vi "Reinitial Parameter After Test.vi"(8 "error in (no error)":errorcluster, 11 "main ref":T1) -> (0 "error out":errorcluster)   [LabVIEW 2025]
uses:
  controls/LAB-IQ UI Data.ctl
  Traction Loop/Traction Receipe Enum.ctl
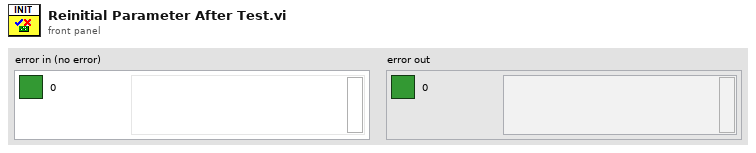
[diagram p1: front panel]
types:
  T1 = typedef "LAB-IQ UI Data.ctl" = cluster{"Main Home Screen":cluster{"GUI":refnum<vi>, "Platform Settings":refnum<vi>, "Configure":refnum<vi>, "Home":refnum<vi>, "EXIT":refnum<vi>, "service 2":refnum<vi>, "MainPage":refnum<vi>, "Analysis":refnum<vi>}, "Platform Settings":cluster{"mm/s  Surge":refnum<vi>, "Drive Error":refnum<vi>, "Disable Axis Jog Soft Limits":refnum<vi>, "mm/s  Sway":refnum<vi>, "Sway and Surge COM Status":refnum<vi>, "Heave COM Status":refnum<vi>, "Enable Platform":refnum<vi>, "Surge Forward Main":refnum<vi>, "Sway Right Main":refnum<vi>, "Sway Left Main":refnum<vi>, "Heave Down Main":refnum<vi>, "Heave Up main":refnum<vi>, "mm/s Heave":refnum<vi>, "mm/sec":refnum<vi>, "mm":refnum<vi>, "Surge Backward Main":refnum<vi>}, "Analysis Screen":cluster{"Analysis Home":refnum<vi>, "Surface Analysis":refnum<vi>, "Imaging":refnum<vi>, "Image Analysis":refnum<vi>, "Post Analysis":refnum<vi>}, "Config Screen":cluster{"Select Load Head":refnum<vi>, "Notes :":refnum<vi>, "FILE":refnum<vi>, "Sample ID :":refnum<vi>, "Operator ID :":refnum<vi>, "Operator Name :":refnum<vi>, "Auto":refnum<vi>}, "Motion Module":cluster{"zNL":refnum<vi>, "NL disp":refnum<vi>, "Rotary Tab":refnum<vi>, "Motion Direction:  3":refnum<vi>, "E.Velocity 2":refnum<vi>, "e.v/ssr 2":refnum<vi>, "Enter Fixed E.Velocity 2":refnum<vi>, "Enter Final SRR 2":refnum<vi>, "Enter initial SRR 2":refnum<vi>, "Enter Fixed SRR 2":refnum<vi>, "Enter the Final E.Velocity (m/s) 2":refnum<vi>, "Enter initial E.Velocity (m/s) 2":refnum<vi>, "Final Speed (RPM) 3":refnum<vi>, "Initial Speed (RPM) 2":refnum<vi>, "Enter the Final Velocity (m/s) 3":refnum<vi>, "Enter initial Velocity (m/s)  3":refnum<vi>, "Ramp Up 2":refnum<vi>, "TEST SELECTION":refnum<vi>, "SPEED SELECTION : ":refnum<vi>, "Angular Oscillation Set":refnum<vi>, "Traction":refnum<vi>, "Step Speed":refnum<vi>, "StepTable For Load-Speed":refnum<vi>, "StepTable For Speed":refnum<vi>, "Surge Forward MM":refnum<vi>, "Surge Backward MM":refnum<vi>, "M3 Image":refnum<vi>, "String 39":refnum<vi>, "Sway Left MM":refnum<vi>, "Sway Right MM":refnum<vi>, "Disable Axis Jog Soft Limits":refnum<vi>, "mm":refnum<vi>, "Heave Down MM":refnum<vi>, "Heave Up MM":refnum<vi>, "Wear Track Diameter (mm)":refnum<vi>, "Set WTD":refnum<vi>, "HomeScratch":refnum<vi>, "HomeRot":refnum<vi>, "PlaceModule":refnum<vi>, "Enter the Angle (Deg)":refnum<vi>, "Enter the Frequency (Hz)":refnum<vi>, "Motion Mode:":refnum<vi>, "LR Sway":refnum<vi>, "Rot Hor":refnum<vi>, "Scratch":refnum<vi>, "LR Cam":refnum<vi>, "MMBack":refnum<vi>, "MMNext":refnum<vi>, "Rot Ver":refnum<vi>, "Rotary Module Selection":refnum<vi>, "calculate rotary":refnum<vi>, "SPEED SELECTION : rotary":refnum<vi>, "Import 2":refnum<vi>, "Save 2":refnum<vi>, "File Path :  2":refnum<vi>, "String 45":refnum<vi>, "StepTable For Speed 3":refnum<vi>, "Enter the Speed(mm/sec)":refnum<vi>, "Enter the Speed(RPM)":refnum<vi>, "Enter Scratch Speed (mm/s):":refnum<vi>, "SwaySpeed Set":refnum<vi>, "Scartch Offset":refnum<vi>, "Motion type:":refnum<vi>, "HomeScratch 2":refnum<vi>, "Enter Scratch length (mm):":refnum<vi>, "Wear Track Diameter":refnum<vi>, "Rotary Speed Exced":refnum<vi>, "Scratch Mode":refnum<vi>, "No of Scratch":refnum<vi>}, "Environmental control":cluster{"Humidity  Status  3":refnum<vi>, "Low Temp  Status  2":refnum<vi>, "TK4 status 2":refnum<vi>, "Stage Temperature":refnum<vi>, "Sample Temperature":refnum<vi>, "Humidity (Amb)":refnum<vi>, "Clear List":refnum<vi>, "Add to list":refnum<vi>, "Wear":refnum<vi>, "Vibration":refnum<vi>, "Humidity (Chamber)":refnum<vi>, "Temperature (Chamber)":refnum<vi>, "ECR ":refnum<vi>, "Temperature (Amb)":refnum<vi>, "Microphone":refnum<vi>, "Acoustic Emission 3":refnum<vi>, "SNext":refnum<vi>, "APBack":refnum<vi>, "Enter the Temperature (°C):":refnum<vi>, "Enter the Stage \nTemperature (°C):":refnum<vi>, "Enter the Humidity (%Rh):":refnum<vi>, "Low Temp":refnum<vi>, "High Temp":refnum<vi>, "Humidity":refnum<vi>, "Sensors Picked":refnum<vi>}, "About Screen":cluster{"Password":refnum<vi>, "Home Service":refnum<vi>, "Advanced Setting":refnum<vi>, "About Tab":refnum<vi>, "ECR Port:":refnum<vi>, "Ramp Port:":refnum<vi>, "Installation/Replacement completed":refnum<vi>, "Loahead":refnum<vi>, "Heave and Surge COM Port:":refnum<vi>, "Sway COM Port:":refnum<vi>, "Temp Modbus:":refnum<vi>, "Humidity Port:":refnum<vi>, "Edit Gain Constants":refnum<vi>, "Save Gain Constants":refnum<vi>}, "Main Screen":cluster{"Main Screen Tab":refnum<vi>, "Angle and Frequency":refnum<vi>, "Stroke (mm)":refnum<vi>, "Angle (Deg)":refnum<vi>, "Main Speed Tab":refnum<vi>, "MTM MOTOR DISPLAY":refnum<vi>, "Disc Speed (m/sec)":refnum<vi>, "Ball Speed (m/sec)":refnum<vi>, "Disc Speed (RPM)":refnum<vi>, "Ball Speed (RPM)":refnum<vi>, "SPEED TAB":refnum<vi>, "Speed (m/sec)":refnum<vi>, "Set Speed (m/sec)":refnum<vi>, "Speed (RPM)":refnum<vi>, "Set Speed":refnum<vi>, "Time Tab":refnum<vi>, "Time ( HH:MM:SS ) 2":refnum<vi>, "Test Duration":refnum<vi>, "Test Duration 4":refnum<vi>, "TEST CYCLE":refnum<vi>, "TOTAL CYCLES":refnum<vi>, "Set Load (N)":refnum<vi>, "Temp Tabs":refnum<vi>, "Heater":refnum<vi>, "TK4 status":refnum<vi>, "ChamberTemp":refnum<vi>, "SetTmp":refnum<vi>, "Controller  Status":refnum<vi>, "ChamberTemp 2":refnum<vi>, "SetTmp 2":refnum<vi>, "Controller  Status 2":refnum<vi>, "ChamberTemp 3":refnum<vi>, "SetTmp 3":refnum<vi>, "Cooling":refnum<vi>, "Load Communication":refnum<vi>, "Ambient \nTemperature":refnum<vi>, "HumCOMStatus":refnum<vi>, "Ambient\n Humidity":refnum<vi>, "Freq (Hz)":refnum<vi>, "Load En":refnum<vi>, "NLt":refnum<vi>, "zNL 2":refnum<vi>, "Humidity On":refnum<vi>, "humidity disp":refnum<vi>, "Set Humidity":refnum<vi>, "NL disp 2":refnum<vi>, "Humidity On 2":refnum<vi>, "humidity disp 2":refnum<vi>, "Set Humidity 2":refnum<vi>, "NL disp 3":refnum<vi>, "AppLoadSeq scratch":refnum<vi>, "Stop Scratch":refnum<vi>, "ClrLog":refnum<vi>, "Trip Log":refnum<vi>, "STOP":refnum<vi>, "Start Test":refnum<vi>, "Test status":refnum<vi>, "AR Led":refnum<vi>, "Data":refnum<vi>, "Health":refnum<vi>, "Sway COM Status":refnum<vi>, "Heave COM Status":refnum<vi>, "Grp Tab":refnum<vi>, "Sub Graph":refnum<vi>, "SD (mm)":refnum<vi>, "Siliding distance Reset Graph":refnum<vi>, "SDGp":refnum<vi>, "Humidity Reset Graph":refnum<vi>, "HumrGp":refnum<vi>, "Acoustic Emission (mV)":refnum<vi>, "Aqucostic Reset Graph":refnum<vi>, "gACQUOS":refnum<vi>, "ECR RESET":refnum<vi>, "ECR":refnum<vi>, "Temperature Reset":refnum<vi>, "Acoustic Emission (mV) 2":refnum<vi>, "Aqucostic Reset Graph 2":refnum<vi>, "gACQUOS 2":refnum<vi>, "ECR RESET 2":refnum<vi>, "ECR 2":refnum<vi>, "Temperature Reset 2":refnum<vi>, "Temperature (deg c)":refnum<vi>, "Speed Reset Graph":refnum<vi>, "Speed Tab":refnum<vi>, "MTM DISC  SPEED":refnum<vi>, "MTM BALL SPEED":refnum<vi>, "speed mm/sec":refnum<vi>, "Hymidity":refnum<vi>, "Humidity Disable trip":refnum<vi>, "CoF Trip  2":refnum<vi>, "Depth Trip":refnum<vi>, "Weart Deapth":refnum<vi>, "Depth Reset Graph":refnum<vi>, "Weart":refnum<vi>, "Depthz":refnum<vi>, "Depth (µm)":refnum<vi>, "WearGp":refnum<vi>, "NL Trip 2":refnum<vi>, "Load pid":refnum<vi>, "Load Disable Trip":refnum<vi>, "Load Reset Graph":refnum<vi>, "NL Display 4":refnum<vi>, "Main Chart 3":refnum<vi>, "BACK":refnum<vi>, "Depth Trip 2":refnum<vi>, "COF TRIP ":refnum<vi>, "Friction Force (N)":refnum<vi>, "FF Reset Graph":refnum<vi>, "FF Disable Trip":refnum<vi>, "FF TRIP":refnum<vi>, "COF Disable Trip":refnum<vi>, "COF Reset Graph":refnum<vi>, "Start Test Temp":refnum<vi>, "zFF":refnum<vi>, "Friction Force (N) Graph":refnum<vi>, "Coefficient of Friction":refnum<vi>, "Scratch Start Test":refnum<vi>, "FF Tab":refnum<vi>, "Cyclic Friction Force (N)":refnum<vi>, "CZ FF":refnum<vi>, "Cyclic Friction Force (N) Graph":refnum<vi>, "Cyclic Coefficient of Friction":refnum<vi>, "Cyclic FF TRIP":refnum<vi>, "Cyclic FF Disable Trip":refnum<vi>, "cyclic COF Disable Trip":refnum<vi>, "cyclic COF TRIP":refnum<vi>, "cyclic COF Reset Graph":refnum<vi>, "Cyclic FF Reset Graph":refnum<vi>, "Test Trip":refnum<vi>, "Multi Scratch Pass":refnum<vi>, "Scratch Start Recording":refnum<vi>}, "Loading":cluster{"Indentation":refnum<vi>, "Reference Sample":refnum<vi>, "Load Cell Communication Slide":refnum<vi>, "com 3":refnum<vi>, "com":refnum<vi>, "DecaForce COM Status":refnum<vi>, "Update":refnum<vi>, "Clear 3":refnum<vi>, "seq":refnum<vi>, "Stribeck table":refnum<vi>, "Stribeck Table  For loading":refnum<vi>, "Loading Mode":refnum<vi>, "Enter the Final Load (N)":refnum<vi>, "Enter the CoF Trip":refnum<vi>, "Enter the Friction Force Trip":refnum<vi>, "Enter the Normal load Trip":refnum<vi>, "Enter the Load  (N)":refnum<vi>, "KiloForce":refnum<vi>, "DecaForce ":refnum<vi>, "MicroForce":refnum<vi>, "LHBack":refnum<vi>, "LHNext":refnum<vi>, "Enter the Loading Rate (N/min)":refnum<vi>, "Message":refnum<vi>, "Warning 2":refnum<vi>, "SSP 0.75":refnum<vi>, "SSP 0.5":refnum<vi>, "SSP 0.3":refnum<vi>, "Warning":refnum<vi>, "gui GIF":refnum<vi>, "Communication is established":refnum<vi>, "AppLoad 4":refnum<vi>, "Multipoint":refnum<vi>, "Load Selection":refnum<vi>}, "PID":cluster{"Ramp":refnum<vi>, "Vertical load (N)":refnum<vi>, "apply load":refnum<vi>, "apply load 2":refnum<vi>, "Enter ByPass Load":refnum<vi>, "Bypass Load":refnum<vi>, "gFF Rot":refnum<vi>}, "Config Parameters":cluster{"Tab Control 3":refnum<vi>, "Tab Control 19":refnum<vi>, "SAMPLES":refnum<vi>, "Re-initilaize":refnum<vi>, "Filter ON/OFF":refnum<vi>, "TracHomeSurgeOffsetCounts 10MM":refnum<vi>, "TracHomeSwayOffsetCounts 10MM":refnum<vi>, "Acoustic Emission:":refnum<vi>, "Apply Filter (FF)":refnum<vi>, "Filter% 2":refnum<vi>, "Apply Filter (Load)":refnum<vi>, "Filter% ":refnum<vi>, "Sway distance (mm)":refnum<vi>, "Surge distance (mm)":refnum<vi>, "DataSavingLoopDelay(ms)":refnum<vi>, "SAVE 2":refnum<vi>, "Enter Distance":refnum<vi>, "Sway Counts:":refnum<vi>, "Distance (mm): 3":refnum<vi>, "Surge Counts:":refnum<vi>, "Distance (mm): 2":refnum<vi>, "Distance (mm):":refnum<vi>, "Heave Counts:":refnum<vi>, "LRMHomeSurgeOffsetCounts":refnum<vi>, "LRMHomeSwayOffsetCounts":refnum<vi>, "TracHomeSurgeOffsetCounts 20MM":refnum<vi>, "TracHomeSwayOffsetCounts 20MM":refnum<vi>, "RotHomeSwayOffsetCounts":refnum<vi>, "RotHomeSurgeOffsetCounts":refnum<vi>, "Heave distance":refnum<vi>, "Zmm":refnum<vi>, "Heave Pulses/mm":refnum<vi>, "Surge Pulses/mm":refnum<vi>, "Sway Pulses/mm":refnum<vi>, "Heave Pitch":refnum<vi>, "Surge Pitch":refnum<vi>, "Sway Pitch":refnum<vi>, "Heave PPR":refnum<vi>, "Surge PPR":refnum<vi>, "Sway PPR":refnum<vi>, "Tab Control 5":refnum<vi>, "Tab Control 14":refnum<vi>, "Tab Control 26":refnum<vi>, "AE":refnum<vi>, "Heave Loop Delay":refnum<vi>, "Heave PID Speed":refnum<vi>, "Surge Jog Speed":refnum<vi>, "Heave Jog Speed":refnum<vi>, "Sway Loop Delay":refnum<vi>, "Sway PID Speed":refnum<vi>, "Sway Jog Speed":refnum<vi>, "DEPTH TRIP VALUE":refnum<vi>, "LOAD TRIP VALUE":refnum<vi>, "DEPTH TRIP   ENABLE":refnum<vi>, "LOAD TRIP  ENABLE":refnum<vi>, "CYCLIC FF TRIP VALUE":refnum<vi>, "FF TRIP VALUE":refnum<vi>, "CYCLIC CoF TRIP VALUE":refnum<vi>, "COF TRIP VALUE":refnum<vi>, "CYCLIC COF TRIP  ENABLE":refnum<vi>, "CYCLIC FF TRIP  ENABLE":refnum<vi>, "FF TRIP  ENABLE":refnum<vi>, "COF TRIP  ENABLE":refnum<vi>, "JOG TRIP LOAD VALUE (N)":refnum<vi>, "Rotary Vertical":refnum<vi>, "Traction":refnum<vi>, "Scratch":refnum<vi>, "LRM CAM":refnum<vi>, "Sway LRM":refnum<vi>, "Rotary Horizontal":refnum<vi>}, "Loading Com Port":cluster{"ClearAll":refnum<vi>, "Mz(Nm)":refnum<vi>, "My(Nm)":refnum<vi>, "Mx(Nm)":refnum<vi>, "Save Dwell":refnum<vi>, "Acq Delay (ms)":refnum<vi>, "Burst Delay (ms)":refnum<vi>, "model":refnum<vi>, "SN":refnum<vi>, "FFx(N)":refnum<vi>, "Sensor IP":refnum<vi>, "Port":refnum<vi>, "FFy(N)":refnum<vi>, "Load(N)":refnum<vi>, "delete Handle":refnum<vi>, "Create Handle":refnum<vi>, "ft_data":refnum<vi>, "ft_range":refnum<vi>, "ft_data 2":refnum<vi>, "stop 6":refnum<vi>, "running_flag":refnum<vi>, "ft_udp_handle":refnum<vi>, "get-data-return":refnum<vi>, "get-range-return":refnum<vi>, "zero-return":refnum<vi>, "filter-return":refnum<vi>, "initial-return":refnum<vi>, "deleteHandle-result":refnum<vi>, "Load Cell Temp":refnum<vi>, "Load Cell":refnum<vi>, "ZeroAll":refnum<vi>, "FORCE (N)":refnum<vi>, "TORQUE (N-m)":refnum<vi>, "Load Cell Link":refnum<vi>}, "Heave AND Surge":cluster{"SURGE POSE":refnum<vi>, "error out Read":refnum<vi>, "HEAVE POSE":refnum<vi>, "State":refnum<vi>, "Homed":refnum<vi>, "Sequence ID":refnum<vi>, "error out Write":refnum<vi>, "faultCode":refnum<vi>, "Ack ID":refnum<vi>, "SPEED":refnum<vi>, "Distance":refnum<vi>, "Mode Command":refnum<vi>, "Heave and Surge Read":refnum<vi>, "Read Heave Temp":refnum<vi>, "Spare 15":refnum<vi>, "Spare 14":refnum<vi>, "Spare 13":refnum<vi>, "Spare 12":refnum<vi>, "Spare 11":refnum<vi>, "Spare 10":refnum<vi>, "Spare 9":refnum<vi>, "Spare 8":refnum<vi>, "Spare 7":refnum<vi>, "Spare 4":refnum<vi>, "Spare 3":refnum<vi>, "Spare 2":refnum<vi>, "Humidity":refnum<vi>, "Temp":refnum<vi>, "Node Id":refnum<vi>, "Spare 1":refnum<vi>, "SPARE 4":refnum<vi>, "SPARE 3":refnum<vi>, "SPARE 2":refnum<vi>, "SPARE 1":refnum<vi>, "fwMajor":refnum<vi>, "fwMinor":refnum<vi>, "Manual Write":refnum<vi>, "Heave and Surge Write":refnum<vi>, "SPARE 5":refnum<vi>, "Reserved ":refnum<vi>, "SPARE 8":refnum<vi>, "SPARE 6":refnum<vi>, "SPARE 7":refnum<vi>, "SPARE 17":refnum<vi>, "SPARE 16":refnum<vi>, "SPARE 15":refnum<vi>, "SPARE 14":refnum<vi>, "SPARE 13":refnum<vi>, "SPARE 12":refnum<vi>, "SPARE 11":refnum<vi>, "SPARE 10":refnum<vi>, "SPARE 9":refnum<vi>, "System UPTIME":refnum<vi>, "Missed Packets":refnum<vi>, "faultCode Surge Right":refnum<vi>, "faultCode Surge Left":refnum<vi>, "faultCode Heave":refnum<vi>, "UPLINK HEAVE":refnum<vi>, "DOWNLINK HEAVE":refnum<vi>}, "New PID LOGIC":cluster{"Fine Tune Zone":refnum<vi>, "PID SDelay":refnum<vi>, "Max_pos_limit":refnum<vi>, "Min_pos_limit":refnum<vi>, "i_limit":refnum<vi>, "pct_scale":refnum<vi>, "Deadband":refnum<vi>, "Kd":refnum<vi>, "Ki":refnum<vi>, "Kp":refnum<vi>, "Current Position":refnum<vi>, "Set Load":refnum<vi>, "Current Load":refnum<vi>, "Pulse delta":refnum<vi>, "Init Step":refnum<vi>, "Max Step Linit":refnum<vi>, "min_deadband_floor":refnum<vi>, "dynamic_spindle_noise_scalar":refnum<vi>, "min_finetune_floor":refnum<vi>, "filter_alpha":refnum<vi>, "PID":refnum<vi>}, "SWAY ":cluster{"fwMajor":refnum<vi>, "Homed":refnum<vi>, "Rotary POSE":refnum<vi>, "State":refnum<vi>, "SWAY POSE":refnum<vi>, "Ack ID":refnum<vi>, "faultCode":refnum<vi>, "Node Id":refnum<vi>, "fwMinor":refnum<vi>, "Spare 6":refnum<vi>, "Spare 5":refnum<vi>, "Spare 4":refnum<vi>, "Spare 3":refnum<vi>, "Spare 2":refnum<vi>, "Spare 1":refnum<vi>, "Spare 7":refnum<vi>, "SPARE  5":refnum<vi>, "error out Write  SWAY ":refnum<vi>, "error out Read SWAY ":refnum<vi>, "Manual Write SWAY ":refnum<vi>, "SWAY WRITE":refnum<vi>, "SPARE  4":refnum<vi>, "SPARE  3":refnum<vi>, "SPARE 2":refnum<vi>, "SPARE 1":refnum<vi>, "Spare 15":refnum<vi>, "Spare 14":refnum<vi>, "Spare 13":refnum<vi>, "Spare 12":refnum<vi>, "Spare 11":refnum<vi>, "Spare 9":refnum<vi>, "Spare 8":refnum<vi>, "SPEED":refnum<vi>, "Distance":refnum<vi>, "Mode Command":refnum<vi>, "Sequence ID":refnum<vi>, "SWAY READ":refnum<vi>, "Spare 10":refnum<vi>, "Read SWAY Temp":refnum<vi>, "faultCode Sway ":refnum<vi>, "Missed Packets":refnum<vi>, "System UPTIME sway":refnum<vi>, "SPARE 6":refnum<vi>, "SPARE 7":refnum<vi>, "SPARE 9":refnum<vi>, "SPARE 11":refnum<vi>, "SPARE 10":refnum<vi>, "SPARE 8":refnum<vi>, "SPARE 13":refnum<vi>, "SPARE 12":refnum<vi>, "SPARE 17":refnum<vi>, "SPARE 16":refnum<vi>, "SPARE 15":refnum<vi>, "SPARE 14":refnum<vi>, "Reserved":refnum<vi>, "faultCode Rotary":refnum<vi>, "UPLINK SWAY":refnum<vi>, "DOWNLINK SWAY":refnum<vi>}, "Analysis Screen":cluster{"Analysis Home":refnum<vi>, "Refresh 2":refnum<vi>, "MEAN 4":refnum<vi>, "SD 4":refnum<vi>, "VARIANCE 4":refnum<vi>, "MEAN  3":refnum<vi>, "SD  3":refnum<vi>, "VARIANCE  3":refnum<vi>, "MEAN 2":refnum<vi>, "SD  2":refnum<vi>, "VARIANCE 2":refnum<vi>, "MEAN":refnum<vi>, "SD":refnum<vi>, "VARIANCE":refnum<vi>, "File 4 Discription":refnum<vi>, "OPEN 4":refnum<vi>, "File Name 4":refnum<vi>, "OPEN 3":refnum<vi>, "File 3 Discription":refnum<vi>, "File Name 3":refnum<vi>, "Y-AXIS":refnum<vi>, "X-AXIS":refnum<vi>, "XY Graph":refnum<vi>, "File Name 2":refnum<vi>, "File Name 1":refnum<vi>, "OPEN 2":refnum<vi>, "OPEN 1":refnum<vi>, "File 1 Discription ":refnum<vi>, "File 2 Discription":refnum<vi>, "Export":refnum<vi>, "File Format":refnum<vi>}, "Traction":cluster{"faultCode Traction 2":refnum<vi>, "faultCode Traction 1":refnum<vi>, "Missed Packets":refnum<vi>, "System UPTIME Traction":refnum<vi>, "SPARE 17":refnum<vi>, "SPARE 16":refnum<vi>, "SPARE 15":refnum<vi>, "SPARE 14":refnum<vi>, "SPARE 13":refnum<vi>, "SPARE 12":refnum<vi>, "SPARE 11":refnum<vi>, "SPARE 10":refnum<vi>, "SPARE 9":refnum<vi>, "SPARE 8":refnum<vi>, "SPARE 7":refnum<vi>, "SPARE 6":refnum<vi>, "Reserved":refnum<vi>, "SPARE  5":refnum<vi>, "Manual Write TRACTION":refnum<vi>, "TRACTION WRITE":refnum<vi>, "SPARE  4":refnum<vi>, "SPARE  3":refnum<vi>, "SPARE 2":refnum<vi>, "SPARE 1":refnum<vi>, "Spare 7":refnum<vi>, "Spare 6":refnum<vi>, "Spare 5":refnum<vi>, "Spare 4":refnum<vi>, "Spare 2":refnum<vi>, "Spare 1":refnum<vi>, "Node Id":refnum<vi>, "Read TRACTION Temp":refnum<vi>, "fwMinor":refnum<vi>, "fwMajor":refnum<vi>, "faultCode":refnum<vi>, "TRACTION POSE":refnum<vi>, "TRACTION POSE 2":refnum<vi>, "Homed":refnum<vi>, "State":refnum<vi>, "Ack ID":refnum<vi>, "SPEED":refnum<vi>, "Distance":refnum<vi>, "Mode Command":refnum<vi>, "Sequence ID":refnum<vi>, "error out Read TRACTION":refnum<vi>, "error out Write  TRACTION":refnum<vi>, "TRACTION READ":refnum<vi>, "Spare 3":refnum<vi>, "Downlink traction":refnum<vi>, "Uplink Traction":refnum<vi>}, "Traction reciepe":cluster{"SRR Sweep Range (%) Stribeck":refnum<vi>, "Traction Receipe":refnum<vi>, "Total Execution Time":refnum<vi>, "Total Steps":refnum<vi>, "Duration / Step (s)  Stribeck":refnum<vi>, "STRIBECK Fixed SRR List (%)":refnum<vi>, "Duration / Step (s) Traction":refnum<vi>, "SRR Sweep Range (%) traction":refnum<vi>, "Rolling Speed (mm/s)":refnum<vi>, "Temperature Stages (°C)":refnum<vi>, "Ball Load (N)":refnum<vi>, "Lubricant Name":refnum<vi>, "Profile File Name":refnum<vi>, "SET entrainment Velocity":refnum<vi>, "Test Array Size":refnum<vi>, "SRR INDEX [ STRIBECK]":refnum<vi>, "Stribeck Size":refnum<vi>, "SET SRR":refnum<vi>, "ELAPSED TIMER ":refnum<vi>, "BALL SET RPM":refnum<vi>, "DISC SET RPM":refnum<vi>, "SET LOAD":refnum<vi>, "TEMPERATURE READ":refnum<vi>, "SET TEMPERATURE":refnum<vi>, "Traction Size":refnum<vi>, "DISC SPEED (rpm)":refnum<vi>, "BALL SPEED (rpm)":refnum<vi>, "BALL WEAR TRACK":refnum<vi>, "DISC WEARTRACK":refnum<vi>, "SRR INDEX [ TRACTION]":refnum<vi>, "Start Index Type":refnum<vi>, "Enum - Menu":refnum<vi>, "Ball (mm/sec)":refnum<vi>, "Disc (mm/sec)":refnum<vi>}, "Traction Control":cluster{"HomeTraction":refnum<vi>, "Demo Mode Display":refnum<vi>, "Traction Message":refnum<vi>, "Traction Step Update Details":refnum<vi>, "Main Tab sequence for selection":refnum<vi>, "Ramp Tab":refnum<vi>, "e.v/ssr":refnum<vi>, "Enter Fixed E.Velocity":refnum<vi>, "Enter Final SRR":refnum<vi>, "Enter initial SRR":refnum<vi>, "Enter Fixed SRR":refnum<vi>, "Enter the Final E.Velocity (m/s)":refnum<vi>, "Enter initial E.Velocity (m/s)":refnum<vi>, "Ball WTD":refnum<vi>, "E.Velocity":refnum<vi>, "Enter the Final Velocity (m/s)":refnum<vi>, "Enter initial Velocity (m/s)":refnum<vi>, "Ramp Up   Disc":refnum<vi>, "Initial DiscSpeed (RPM)":refnum<vi>, "Final Speed (RPM) Ball":refnum<vi>, "Final Speed (RPM)":refnum<vi>, "Initial Speed (RPM) Ball":refnum<vi>, "Enter the Final Velocity (m/s) Ball":refnum<vi>, "Enter initial Velocity (m/s) Ball":refnum<vi>, "Ramp Up":refnum<vi>, "ExceedBallSpeed step":refnum<vi>, "ExceedDiscSpeed":refnum<vi>, "BallSpeed Exceed Indication":refnum<vi>, "Apply":refnum<vi>, "SPEED SELECTION : MTM":refnum<vi>, "SPEED SELECTION : MTM 2":refnum<vi>, "TEST SELECTION (MTM)":refnum<vi>, "MTM Test Selection":refnum<vi>, "File Path Tab":refnum<vi>, "File Path String":refnum<vi>, "Save":refnum<vi>, "Save  2":refnum<vi>, "Import ":refnum<vi>, "File Path :":refnum<vi>, "Step Sequence Indication Tab":refnum<vi>, "Step Sequence Indication":refnum<vi>, "Calculate Step":refnum<vi>, "StepTable":refnum<vi>, "ExceedDiscSpeed  Cinstant Speed":refnum<vi>, "ExceedBallSpeed Constant":refnum<vi>, "TEST SELECTION (MTM) 2":refnum<vi>, "SPEED SELECTION : MTM 3":refnum<vi>, "MTM Test Selection 2":refnum<vi>, "Enter the Speed (m/sec): ":refnum<vi>, "Enter the Speed (m/sec):  2":refnum<vi>, "Enter the Speed (RPM):":refnum<vi>, "Lower Spped ":refnum<vi>, "Upper":refnum<vi>, "Enter the Speed (RPM):Ball":refnum<vi>, "Disc Motion Direction: ":refnum<vi>, "Ball Motion Direction :":refnum<vi>, "Motion Mode: ":refnum<vi>, "Wear Track Diameter (mm) ":refnum<vi>, "Disc Speed Indicator":refnum<vi>, "ExceedBallSpeed":refnum<vi>}, "Acquostic":cluster{"Last Config Rejected ":refnum<vi>, "rx command count":refnum<vi>, "Current Filter Id":refnum<vi>, "Isolated Gain":refnum<vi>, "DAQ Status":refnum<vi>, "error out":refnum<vi>, "error in (no error)":refnum<vi>, "Uplink Packet":refnum<vi>, "data out":refnum<vi>, "Downlink Packet":refnum<vi>, "Gains":refnum<vi>, "Manual Write Acquostic":refnum<vi>, "Acoustic Graphs":refnum<vi>}}
  T2 = enum8{"Enabled", "Disabled", "Disabled and Grayed Out"}
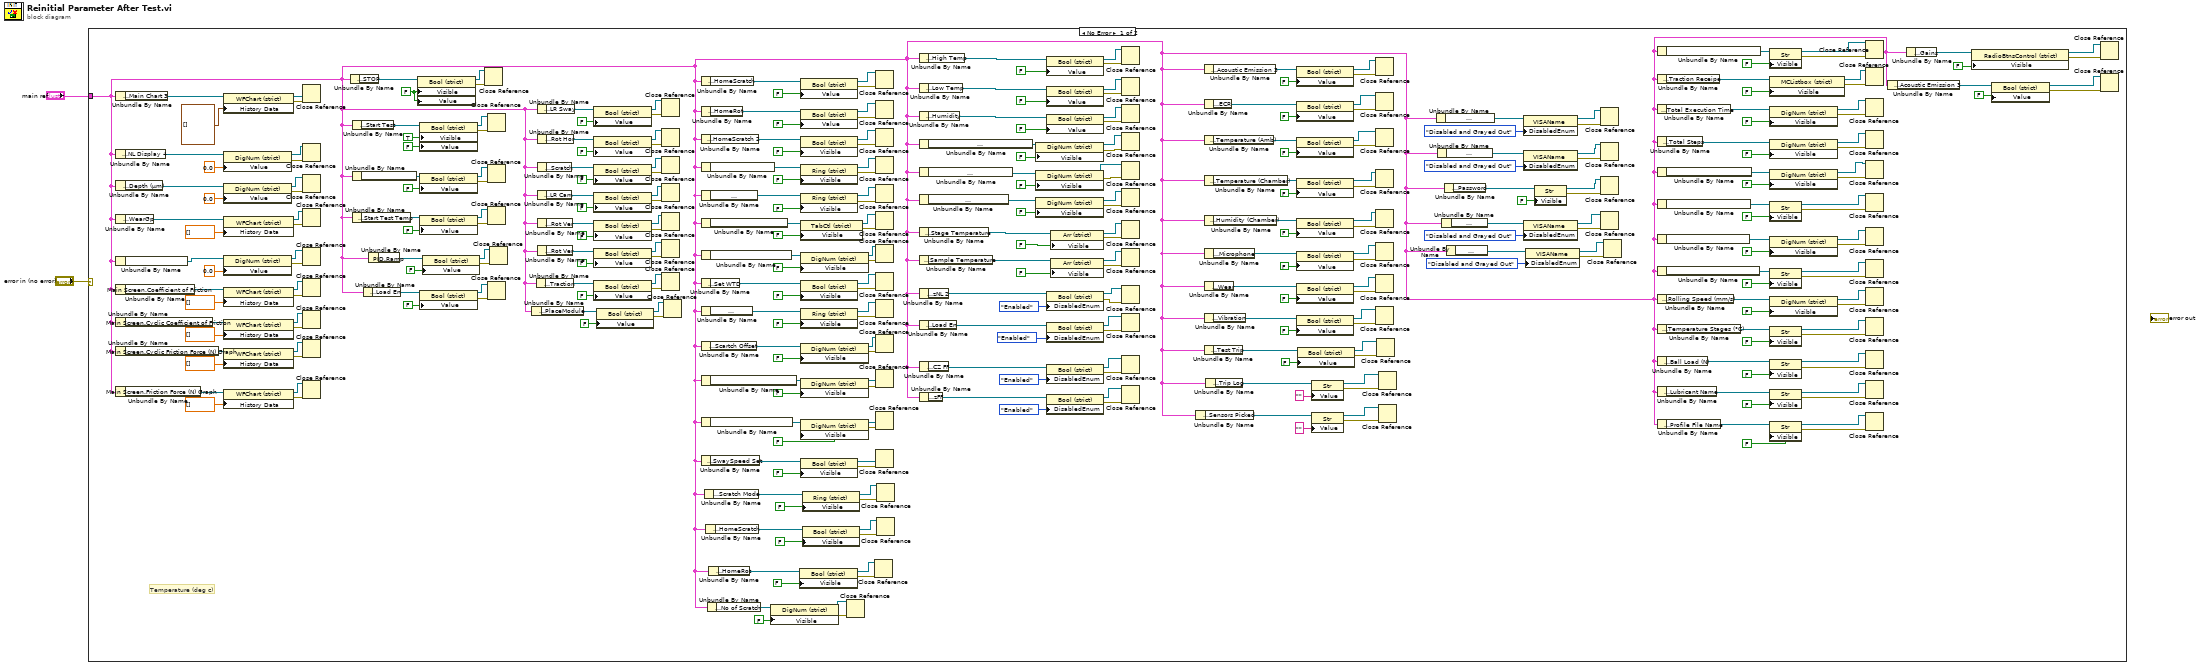
[diagram p0: block diagram]
diagram:
  n1 = case shown="No Error" "error in (no error)" {
    tunnel: "main ref" -> [w4 _]
    frame No Error {
      w285 = FALSE ("Visible")
      # "Temperature (deg c)"
      n2 = Unbundle By Name(w4) -> ("Main Screen.Main Chart 3"=w334:refnum<vi>)
      n3 = Unbundle By Name(w4) -> ("Main Screen.NL Display 4"=w332:refnum<vi>)
      n4 = Unbundle By Name(w4) -> ("Main Screen.Depth (µm)"=w327:refnum<vi>)
      n5 = Unbundle By Name(w4) -> ("Main Screen.WearGp"=w324:refnum<vi>)
      n6 = Unbundle By Name(w4) -> ("Main Screen.Time ( HH:MM:SS ) 2"=w320:refnum<vi>)
      n7 = Unbundle By Name(w4) -> ("Main Screen.Coefficient of Friction"=w317:refnum<vi>)
      n8 = Unbundle By Name(w4) -> ("Main Screen.Cyclic Coefficient of Friction"=w309:refnum<vi>)
      n9 = Unbundle By Name(w4) -> ("Main Screen.Cyclic Friction Force (N) Graph"=w313:refnum<vi>)
      n10 = Unbundle By Name(w4) -> ("Main Screen.Friction Force (N) Graph"=w305:refnum<vi>)
      n11 = property class="WFChart (strict)"(reference=w334, "History Data"=cluster{dbl, "NL disp":dbl, dbl}[] []) -> (reference out=w336:refnum<vi>, error out=w335:errorcluster)  [unwired: 1 in]
      n12 = property class="DigNum (strict)"(reference=w332, "Value"=0.0) -> (reference out=w330:refnum<vi>, error out=w331:errorcluster)  [unwired: 1 in]
      n13 = property class="DigNum (strict)"(reference=w327, "Value"=0.0) -> (reference out=w328:refnum<vi>, error out=w326:errorcluster)  [unwired: 1 in]
      n14 = property class="WFChart (strict)"(reference=w324, "History Data"=dbl[] []) -> (reference out=w322:refnum<vi>, error out=w323:errorcluster)  [unwired: 1 in]
      n15 = property class="DigNum (strict)"(reference=w320, "Value"=0.0) -> (reference out=w301:refnum<vi>, error out=w321:errorcluster)  [unwired: 1 in]
      n16 = property class="WFChart (strict)"(reference=w317, "History Data"=dbl[] []) -> (reference out=w318:refnum<vi>, error out=w316:errorcluster)  [unwired: 1 in]
      n17 = property class="WFChart (strict)"(reference=w309, "History Data"=dbl[] []) -> (reference out=w308:refnum<vi>, error out=w310:errorcluster)  [unwired: 1 in]
      n18 = property class="WFChart (strict)"(reference=w313, "History Data"=dbl[] []) -> (reference out=w311:refnum<vi>, error out=w312:errorcluster)  [unwired: 1 in]
      n19 = property class="WFChart (strict)"(reference=w305, "History Data"=dbl[] []) -> (reference out=w303:refnum<vi>, error out=w304:errorcluster)  [unwired: 1 in]
      n20 = Close Reference(reference=w336, error in (no error)=w335) -> ()  [unwired: 1 out]
      n21 = Close Reference(reference=w330, error in (no error)=w331) -> ()  [unwired: 1 out]
      n22 = Close Reference(reference=w328, error in (no error)=w326) -> ()  [unwired: 1 out]
      n23 = Close Reference(reference=w322, error in (no error)=w323) -> ()  [unwired: 1 out]
      n24 = Close Reference(reference=w301, error in (no error)=w321) -> ()  [unwired: 1 out]
      n25 = Close Reference(reference=w318, error in (no error)=w316) -> ()  [unwired: 1 out]
      n26 = Close Reference(reference=w308, error in (no error)=w310) -> ()  [unwired: 1 out]
      n27 = Close Reference(reference=w311, error in (no error)=w312) -> ()  [unwired: 1 out]
      n28 = Close Reference(reference=w303, error in (no error)=w304) -> ()  [unwired: 1 out]
      n29 = Unbundle By Name(w4) -> ("Main Screen.STOP"=w291:refnum<vi>)
      n30 = Unbundle By Name(w4) -> ("Main Screen.Start Test"=w289:refnum<vi>)
      n31 = Unbundle By Name(w4) -> ("Main Screen.Scratch Start Test"=w297:refnum<vi>)
      n32 = Unbundle By Name(w4) -> ("Main Screen.Start Test Temp"=w298:refnum<vi>)
      n33 = Unbundle By Name(w4) -> ("Main Screen.Load En"=w277:refnum<vi>)
      n34 = Unbundle By Name(w4) -> ("PID.Ramp"=w282:refnum<vi>)
      n35 = property class="Bool (strict)"(reference=w291, "Visible"=w285, "Value"=w285) -> (reference out=w286:refnum<vi>, error out=w292:errorcluster)  [unwired: 1 in]
      n36 = property class="Bool (strict)"(reference=w289, "Visible"=TRUE, "Value"=FALSE) -> (reference out=w287:refnum<vi>, error out=w288:errorcluster)  [unwired: 1 in]
      n37 = property class="Bool (strict)"(reference=w297, "Value"=FALSE) -> (reference out=w295:refnum<vi>, error out=w296:errorcluster)  [unwired: 1 in]
      n38 = property class="Bool (strict)"(reference=w298, "Value"=FALSE) -> (reference out=w300:refnum<vi>, error out=w299:errorcluster)  [unwired: 1 in]
      n39 = property class="Bool (strict)"(reference=w277, "Value"=FALSE) -> (reference out=w279:refnum<vi>, error out=w278:errorcluster)  [unwired: 1 in]
      n40 = property class="Bool (strict)"(reference=w282, "Value"=FALSE) -> (reference out=w280:refnum<vi>, error out=w281:errorcluster)  [unwired: 1 in]
      n41 = Close Reference(reference=w286, error in (no error)=w292) -> ()  [unwired: 1 out]
      n42 = Close Reference(reference=w287, error in (no error)=w288) -> ()  [unwired: 1 out]
      n43 = Close Reference(reference=w295, error in (no error)=w296) -> ()  [unwired: 1 out]
      n44 = Close Reference(reference=w300, error in (no error)=w299) -> ()  [unwired: 1 out]
      n45 = Close Reference(reference=w279, error in (no error)=w278) -> ()  [unwired: 1 out]
      n46 = Close Reference(reference=w280, error in (no error)=w281) -> ()  [unwired: 1 out]
      n47 = Unbundle By Name(w4) -> ("Motion Module.PlaceModule"=w246:refnum<vi>)
      n48 = Unbundle By Name(w4) -> ("Motion Module.Traction"=w250:refnum<vi>)
      n49 = Unbundle By Name(w4) -> ("Motion Module.LR Sway"=w273:refnum<vi>)
      n50 = Unbundle By Name(w4) -> ("Motion Module.Rot Hor"=w270:refnum<vi>)
      n51 = Unbundle By Name(w4) -> ("Motion Module.Scratch"=w266:refnum<vi>)
      n52 = Unbundle By Name(w4) -> ("Motion Module.LR Cam"=w261:refnum<vi>)
      n53 = Unbundle By Name(w4) -> ("Motion Module.Rot Ver"=w258:refnum<vi>)
      n54 = Unbundle By Name(w4) -> ("Motion Module.Rot Ver"=w254:refnum<vi>)
      n55 = property class="Bool (strict)"(reference=w273, "Value"=FALSE) -> (reference out=w275:refnum<vi>, error out=w274:errorcluster)  [unwired: 1 in]
      n56 = property class="Bool (strict)"(reference=w270, "Value"=FALSE) -> (reference out=w268:refnum<vi>, error out=w269:errorcluster)  [unwired: 1 in]
      n57 = property class="Bool (strict)"(reference=w266, "Value"=FALSE) -> (reference out=w264:refnum<vi>, error out=w267:errorcluster)  [unwired: 1 in]
      n58 = property class="Bool (strict)"(reference=w261, "Value"=FALSE) -> (reference out=w263:refnum<vi>, error out=w260:errorcluster)  [unwired: 1 in]
      n59 = property class="Bool (strict)"(reference=w258, "Value"=FALSE) -> (reference out=w256:refnum<vi>, error out=w259:errorcluster)  [unwired: 1 in]
      n60 = property class="Bool (strict)"(reference=w254, "Value"=FALSE) -> (reference out=w252:refnum<vi>, error out=w253:errorcluster)  [unwired: 1 in]
      n61 = property class="Bool (strict)"(reference=w250, "Value"=FALSE) -> (reference out=w248:refnum<vi>, error out=w249:errorcluster)  [unwired: 1 in]
      n62 = property class="Bool (strict)"(reference=w246, "Value"=FALSE) -> (reference out=w244:refnum<vi>, error out=w245:errorcluster)  [unwired: 1 in]
      n63 = Close Reference(reference=w275, error in (no error)=w274) -> ()  [unwired: 1 out]
      n64 = Close Reference(reference=w268, error in (no error)=w269) -> ()  [unwired: 1 out]
      n65 = Close Reference(reference=w264, error in (no error)=w267) -> ()  [unwired: 1 out]
      n66 = Close Reference(reference=w263, error in (no error)=w260) -> ()  [unwired: 1 out]
      n67 = Close Reference(reference=w256, error in (no error)=w259) -> ()  [unwired: 1 out]
      n68 = Close Reference(reference=w252, error in (no error)=w253) -> ()  [unwired: 1 out]
      n69 = Close Reference(reference=w248, error in (no error)=w249) -> ()  [unwired: 1 out]
      n70 = Close Reference(reference=w244, error in (no error)=w245) -> ()  [unwired: 1 out]
      n71 = Unbundle By Name(w4) -> ("Motion Module.HomeScratch"=w214:refnum<vi>)
      n72 = Unbundle By Name(w4) -> ("Motion Module.HomeRot"=w217:refnum<vi>)
      n73 = Unbundle By Name(w4) -> ("Motion Module.HomeScratch 2"=w221:refnum<vi>)
      n74 = Unbundle By Name(w4) -> ("Motion Module.Motion Direction:  3"=w226:refnum<vi>)
      n75 = Unbundle By Name(w4) -> ("Motion Module.Motion Mode:"=w229:refnum<vi>)
      n76 = Unbundle By Name(w4) -> ("Motion Module.Rotary Module Selection"=w233:refnum<vi>)
      n77 = Unbundle By Name(w4) -> ("Motion Module.Wear Track Diameter (mm)"=w237:refnum<vi>)
      n78 = Unbundle By Name(w4) -> ("Motion Module.Set WTD"=w241:refnum<vi>)
      n79 = Unbundle By Name(w4) -> ("Motion Module.Motion type:"=w210:refnum<vi>)
      n80 = Unbundle By Name(w4) -> ("Motion Module.Scartch Offset"=w207:refnum<vi>)
      n81 = Unbundle By Name(w4) -> ("Motion Module.Enter Scratch Speed (mm/s):"=w202:refnum<vi>)
      n82 = Unbundle By Name(w4) -> ("Motion Module.Enter Scratch length (mm):"=w198:refnum<vi>)
      n83 = Unbundle By Name(w4) -> ("Motion Module.SwaySpeed Set"=w194:refnum<vi>)
      n84 = Unbundle By Name(w4) -> ("Motion Module.Scratch Mode"=w143:refnum<vi>)
      n85 = Unbundle By Name(w4) -> ("Motion Module.HomeScratch"=w138:refnum<vi>)
      n86 = Unbundle By Name(w4) -> ("Motion Module.No of Scratch"=w66:refnum<vi>)
      n87 = Unbundle By Name(w4) -> ("Motion Module.HomeRot"=w135:refnum<vi>)
      n88 = property class="DigNum (strict)"(reference=w66, "Visible"=FALSE) -> (reference out=w67:refnum<vi>, error out=w65:errorcluster)  [unwired: 1 in]
      n89 = property class="Bool (strict)"(reference=w135, "Visible"=FALSE ("Value")) -> (reference out=w133:refnum<vi>, error out=w136:errorcluster)  [unwired: 1 in]
      n90 = property class="Bool (strict)"(reference=w214, "Value"=FALSE) -> (reference out=w212:refnum<vi>, error out=w213:errorcluster)  [unwired: 1 in]
      n91 = property class="Bool (strict)"(reference=w217, "Value"=FALSE) -> (reference out=w219:refnum<vi>, error out=w218:errorcluster)  [unwired: 1 in]
      n92 = property class="Bool (strict)"(reference=w221, "Visible"=FALSE ("Value")) -> (reference out=w223:refnum<vi>, error out=w220:errorcluster)  [unwired: 1 in]
      n93 = property class="Ring (strict)"(reference=w226, "Visible"=FALSE ("Value")) -> (reference out=w224:refnum<vi>, error out=w227:errorcluster)  [unwired: 1 in]
      n94 = property class="Ring (strict)"(reference=w229, "Visible"=FALSE ("Value")) -> (reference out=w231:refnum<vi>, error out=w228:errorcluster)  [unwired: 1 in]
      n95 = property class="TabCtl (strict)"(reference=w233, "Visible"=FALSE ("Value")) -> (reference out=w235:refnum<vi>, error out=w234:errorcluster)  [unwired: 1 in]
      n96 = property class="DigNum (strict)"(reference=w237, "Visible"=FALSE ("Value")) -> (reference out=w239:refnum<vi>, error out=w238:errorcluster)  [unwired: 1 in]
      n97 = property class="Bool (strict)"(reference=w241, "Visible"=FALSE ("Value")) -> (reference out=w243:refnum<vi>, error out=w242:errorcluster)  [unwired: 1 in]
      n98 = property class="Ring (strict)"(reference=w210, "Visible"=FALSE ("Value")) -> (reference out=w205:refnum<vi>, error out=w209:errorcluster)  [unwired: 1 in]
      n99 = property class="DigNum (strict)"(reference=w207, "Visible"=FALSE ("Value")) -> (reference out=w204:refnum<vi>, error out=w206:errorcluster)  [unwired: 1 in]
      n100 = property class="DigNum (strict)"(reference=w202, "Visible"=FALSE ("Value")) -> (reference out=w200:refnum<vi>, error out=w201:errorcluster)  [unwired: 1 in]
      n101 = property class="DigNum (strict)"(reference=w198, "Visible"=FALSE ("Value")) -> (reference out=w196:refnum<vi>, error out=w197:errorcluster)  [unwired: 1 in]
      n102 = property class="Bool (strict)"(reference=w194, "Visible"=FALSE ("Value")) -> (reference out=w192:refnum<vi>, error out=w193:errorcluster)  [unwired: 1 in]
      n103 = property class="Ring (strict)"(reference=w143, "Visible"=FALSE ("Value")) -> (reference out=w141:refnum<vi>, error out=w144:errorcluster)  [unwired: 1 in]
      n104 = property class="Bool (strict)"(reference=w138, "Visible"=FALSE ("Value")) -> (reference out=w140:refnum<vi>, error out=w137:errorcluster)  [unwired: 1 in]
      n105 = Close Reference(reference=w67, error in (no error)=w65) -> ()  [unwired: 1 out]
      n106 = Close Reference(reference=w133, error in (no error)=w136) -> ()  [unwired: 1 out]
      n107 = Close Reference(reference=w212, error in (no error)=w213) -> ()  [unwired: 1 out]
      n108 = Close Reference(reference=w219, error in (no error)=w218) -> ()  [unwired: 1 out]
      n109 = Close Reference(reference=w223, error in (no error)=w220) -> ()  [unwired: 1 out]
      n110 = Close Reference(reference=w224, error in (no error)=w227) -> ()  [unwired: 1 out]
      n111 = Close Reference(reference=w231, error in (no error)=w228) -> ()  [unwired: 1 out]
      n112 = Close Reference(reference=w235, error in (no error)=w234) -> ()  [unwired: 1 out]
      n113 = Close Reference(reference=w239, error in (no error)=w238) -> ()  [unwired: 1 out]
      n114 = Close Reference(reference=w243, error in (no error)=w242) -> ()  [unwired: 1 out]
      n115 = Close Reference(reference=w205, error in (no error)=w209) -> ()  [unwired: 1 out]
      n116 = Close Reference(reference=w204, error in (no error)=w206) -> ()  [unwired: 1 out]
      n117 = Close Reference(reference=w200, error in (no error)=w201) -> ()  [unwired: 1 out]
      n118 = Close Reference(reference=w196, error in (no error)=w197) -> ()  [unwired: 1 out]
      n119 = Close Reference(reference=w192, error in (no error)=w193) -> ()  [unwired: 1 out]
      n120 = Close Reference(reference=w141, error in (no error)=w144) -> ()  [unwired: 1 out]
      n121 = Close Reference(reference=w140, error in (no error)=w137) -> ()  [unwired: 1 out]
      n122 = Unbundle By Name(w4) -> ("Environmental control.High Temp"=w162:refnum<vi>)
      n123 = Unbundle By Name(w4) -> ("Environmental control.Low Temp"=w165:refnum<vi>)
      n124 = Unbundle By Name(w4) -> ("Environmental control.Humidity"=w169:refnum<vi>)
      n125 = Unbundle By Name(w4) -> ("Environmental control.Enter the Stage \nTemperature (°C):"=w174:refnum<vi>)
      n126 = Unbundle By Name(w4) -> ("Environmental control.Enter the Temperature (°C):"=w177:refnum<vi>)
      n127 = Unbundle By Name(w4) -> ("Environmental control.Enter the Humidity (%Rh):"=w181:refnum<vi>)
      n128 = Unbundle By Name(w4) -> ("Environmental control.Stage Temperature"=w185:refnum<vi>)
      n129 = Unbundle By Name(w4) -> ("Environmental control.Sample Temperature"=w189:refnum<vi>)
      n130 = Unbundle By Name(w4) -> ("Main Screen.zNL 2"=w160:refnum<vi>)
      n131 = Unbundle By Name(w4) -> ("Main Screen.Load En"=w156:refnum<vi>)
      n132 = Unbundle By Name(w4) -> ("Main Screen.CZ FF"=w150:refnum<vi>)
      n133 = Unbundle By Name(w4) -> ("Main Screen.zFF"=w147:refnum<vi>)
      n134 = property class="DigNum (strict)"(reference=w174, "Visible"=FALSE ("Value")) -> (reference out=w172:refnum<vi>, error out=w175:errorcluster)  [unwired: 1 in]
      n135 = property class="DigNum (strict)"(reference=w177, "Visible"=FALSE ("Value")) -> (reference out=w179:refnum<vi>, error out=w176:errorcluster)  [unwired: 1 in]
      n136 = property class="DigNum (strict)"(reference=w181, "Visible"=FALSE ("Value")) -> (reference out=w183:refnum<vi>, error out=w182:errorcluster)  [unwired: 1 in]
      n137 = property class="Bool (strict)"(reference=w162, "Value"=FALSE) -> (reference out=w132:refnum<vi>, error out=w161:errorcluster)  [unwired: 1 in]
      n138 = property class="Bool (strict)"(reference=w165, "Value"=FALSE) -> (reference out=w167:refnum<vi>, error out=w166:errorcluster)  [unwired: 1 in]
      n139 = property class="Bool (strict)"(reference=w169, "Value"=FALSE) -> (reference out=w171:refnum<vi>, error out=w168:errorcluster)  [unwired: 1 in]
      n140 = property class="Bool (strict)"(reference=w160, "DisabledEnum"=T2."Enabled" ("Disabled")) -> (reference out=w158:refnum<vi>, error out=w159:errorcluster)  [unwired: 1 in]
      n141 = property class="Bool (strict)"(reference=w156, "DisabledEnum"=T2."Enabled" ("Disabled")) -> (reference out=w154:refnum<vi>, error out=w155:errorcluster)  [unwired: 1 in]
      n142 = property class="Bool (strict)"(reference=w150, "DisabledEnum"=T2."Enabled" ("Disabled")) -> (reference out=w149:refnum<vi>, error out=w151:errorcluster)  [unwired: 1 in]
      n143 = property class="Bool (strict)"(reference=w147, "DisabledEnum"=T2."Enabled" ("Disabled")) -> (reference out=w148:refnum<vi>, error out=w146:errorcluster)  [unwired: 1 in]
      n144 = property class="Arr (strict)"(reference=w185, "Visible"=FALSE ("Value")) -> (reference out=w187:refnum<vi>, error out=w186:errorcluster)  [unwired: 1 in]
      n145 = property class="Arr (strict)"(reference=w189, "Visible"=FALSE ("Value")) -> (reference out=w191:refnum<vi>, error out=w190:errorcluster)  [unwired: 1 in]
      n146 = Close Reference(reference=w132, error in (no error)=w161) -> ()  [unwired: 1 out]
      n147 = Close Reference(reference=w167, error in (no error)=w166) -> ()  [unwired: 1 out]
      n148 = Close Reference(reference=w171, error in (no error)=w168) -> ()  [unwired: 1 out]
      n149 = Close Reference(reference=w172, error in (no error)=w175) -> ()  [unwired: 1 out]
      n150 = Close Reference(reference=w179, error in (no error)=w176) -> ()  [unwired: 1 out]
      n151 = Close Reference(reference=w183, error in (no error)=w182) -> ()  [unwired: 1 out]
      n152 = Close Reference(reference=w187, error in (no error)=w186) -> ()  [unwired: 1 out]
      n153 = Close Reference(reference=w191, error in (no error)=w190) -> ()  [unwired: 1 out]
      n154 = Close Reference(reference=w158, error in (no error)=w159) -> ()  [unwired: 1 out]
      n155 = Close Reference(reference=w154, error in (no error)=w155) -> ()  [unwired: 1 out]
      n156 = Close Reference(reference=w149, error in (no error)=w151) -> ()  [unwired: 1 out]
      n157 = Close Reference(reference=w148, error in (no error)=w146) -> ()  [unwired: 1 out]
      n158 = Unbundle By Name(w4) -> ("Environmental control.Sensors Picked"=w89:refnum<vi>)
      n159 = Unbundle By Name(w4) -> ("Environmental control.Acoustic Emission 3"=w130:refnum<vi>)
      n160 = Unbundle By Name(w4) -> ("Environmental control.ECR"=w126:refnum<vi>)
      n161 = Unbundle By Name(w4) -> ("Environmental control.Temperature (Amb)"=w124:refnum<vi>)
      n162 = Unbundle By Name(w4) -> ("Environmental control.Temperature (Chamber)"=w121:refnum<vi>)
      n163 = Unbundle By Name(w4) -> ("Environmental control.Humidity (Chamber)"=w118:refnum<vi>)
      n164 = Unbundle By Name(w4) -> ("Environmental control.Microphone"=w115:refnum<vi>)
      n165 = Unbundle By Name(w4) -> ("Environmental control.Wear"=w112:refnum<vi>)
      n166 = Unbundle By Name(w4) -> ("Environmental control.Vibration"=w109:refnum<vi>)
      n167 = Unbundle By Name(w4) -> ("Main Screen.Test Trip"=w98:refnum<vi>)
      n168 = Unbundle By Name(w4) -> ("Main Screen.Trip Log"=w94:refnum<vi>)
      n169 = property class="Bool (strict)"(reference=w130, "Value"=FALSE) -> (reference out=w131:refnum<vi>, error out=w129:errorcluster)  [unwired: 1 in]
      n170 = property class="Bool (strict)"(reference=w126, "Value"=FALSE) -> (reference out=w128:refnum<vi>, error out=w127:errorcluster)  [unwired: 1 in]
      n171 = property class="Bool (strict)"(reference=w124, "Value"=FALSE) -> (reference out=w123:refnum<vi>, error out=w125:errorcluster)  [unwired: 1 in]
      n172 = property class="Bool (strict)"(reference=w121, "Value"=FALSE) -> (reference out=w122:refnum<vi>, error out=w120:errorcluster)  [unwired: 1 in]
      n173 = property class="Bool (strict)"(reference=w118, "Value"=FALSE) -> (reference out=w117:refnum<vi>, error out=w119:errorcluster)  [unwired: 1 in]
      n174 = property class="Bool (strict)"(reference=w115, "Value"=FALSE) -> (reference out=w116:refnum<vi>, error out=w114:errorcluster)  [unwired: 1 in]
      n175 = property class="Bool (strict)"(reference=w112, "Value"=FALSE) -> (reference out=w111:refnum<vi>, error out=w113:errorcluster)  [unwired: 1 in]
      n176 = property class="Bool (strict)"(reference=w109, "Value"=FALSE) -> (reference out=w110:refnum<vi>, error out=w108:errorcluster)  [unwired: 1 in]
      n177 = property class="Bool (strict)"(reference=w98, "Value"=FALSE) -> (reference out=w99:refnum<vi>, error out=w97:errorcluster)  [unwired: 1 in]
      n178 = property class="Str"(reference=w94, "Value"="") -> (reference out=w93:refnum<vi>, error out=w95:errorcluster)  [unwired: 1 in]
      n179 = property class="Str"(reference=w89, "Value"="") -> (reference out=w90:refnum<vi>, error out=w88:errorcluster)  [unwired: 1 in]
      n180 = Close Reference(reference=w131, error in (no error)=w129) -> ()  [unwired: 1 out]
      n181 = Close Reference(reference=w128, error in (no error)=w127) -> ()  [unwired: 1 out]
      n182 = Close Reference(reference=w123, error in (no error)=w125) -> ()  [unwired: 1 out]
      n183 = Close Reference(reference=w122, error in (no error)=w120) -> ()  [unwired: 1 out]
      n184 = Close Reference(reference=w117, error in (no error)=w119) -> ()  [unwired: 1 out]
      n185 = Close Reference(reference=w116, error in (no error)=w114) -> ()  [unwired: 1 out]
      n186 = Close Reference(reference=w111, error in (no error)=w113) -> ()  [unwired: 1 out]
      n187 = Close Reference(reference=w110, error in (no error)=w108) -> ()  [unwired: 1 out]
      n188 = Close Reference(reference=w99, error in (no error)=w97) -> ()  [unwired: 1 out]
      n189 = Close Reference(reference=w93, error in (no error)=w95) -> ()  [unwired: 1 out]
      n190 = Close Reference(reference=w90, error in (no error)=w88) -> ()  [unwired: 1 out]
      n191 = Unbundle By Name(w4) -> ("About Screen.Temp Modbus:"=w86:refnum<vi>)
      n192 = Unbundle By Name(w4) -> ("About Screen.Humidity Port:"=w85:refnum<vi>)
      n193 = Unbundle By Name(w4) -> ("About Screen.Ramp Port:"=w73:refnum<vi>)
      n194 = Unbundle By Name(w4) -> ("About Screen.Password"=w80:refnum<vi>)
      n195 = Unbundle By Name(w4) -> ("About Screen.ECR Port:"=w72:refnum<vi>)
      n196 = property class="VISAName"(reference=w86, "DisabledEnum"=T2."Disabled and Grayed Out" ("Disabled")) -> (reference out=w76:refnum<vi>, error out=w87:errorcluster)  [unwired: 1 in]
      n197 = property class="VISAName"(reference=w85, "DisabledEnum"=T2."Disabled and Grayed Out" ("Disabled")) -> (reference out=w83:refnum<vi>, error out=w84:errorcluster)  [unwired: 1 in]
      n198 = property class="VISAName"(reference=w73, "DisabledEnum"=T2."Disabled and Grayed Out" ("Disabled")) -> (reference out=w68:refnum<vi>, error out=w74:errorcluster)  [unwired: 1 in]
      n199 = property class="VISAName"(reference=w72, "DisabledEnum"=T2."Disabled and Grayed Out" ("Disabled")) -> (reference out=w69:refnum<vi>, error out=w71:errorcluster)  [unwired: 1 in]
      n200 = property class="Str"(reference=w80, "Visible"=FALSE) -> (reference out=w82:refnum<vi>, error out=w81:errorcluster)  [unwired: 1 in]
      n201 = Close Reference(reference=w76, error in (no error)=w87) -> ()  [unwired: 1 out]
      n202 = Close Reference(reference=w83, error in (no error)=w84) -> ()  [unwired: 1 out]
      n203 = Close Reference(reference=w82, error in (no error)=w81) -> ()  [unwired: 1 out]
      n204 = Close Reference(reference=w68, error in (no error)=w74) -> ()  [unwired: 1 out]
      n205 = Close Reference(reference=w69, error in (no error)=w71) -> ()  [unwired: 1 out]
      n206 = Unbundle By Name(w4) -> ("Traction reciepe.SRR Sweep Range (%) Stribeck"=w46:refnum<vi>)
      n207 = Unbundle By Name(w4) -> ("Traction reciepe.Traction Receipe"=w49:refnum<vi>)
      n208 = Unbundle By Name(w4) -> ("Traction reciepe.Total Execution Time"=w52:refnum<vi>)
      n209 = Unbundle By Name(w4) -> ("Traction reciepe.Total Steps"=w44:refnum<vi>)
      n210 = Unbundle By Name(w4) -> ("Traction reciepe.Duration / Step (s)  Stribeck"=w41:refnum<vi>)
      n211 = Unbundle By Name(w4) -> ("Traction reciepe.STRIBECK Fixed SRR List (%)"=w38:refnum<vi>)
      n212 = Unbundle By Name(w4) -> ("Traction reciepe.Duration / Step (s) Traction"=w61:refnum<vi>)
      n213 = Unbundle By Name(w4) -> ("Traction reciepe.SRR Sweep Range (%) traction"=w25:refnum<vi>)
      n214 = Unbundle By Name(w4) -> ("Traction reciepe.Rolling Speed (mm/s)"=w22:refnum<vi>)
      n215 = Unbundle By Name(w4) -> ("Traction reciepe.Temperature Stages (°C)"=w19:refnum<vi>)
      n216 = Unbundle By Name(w4) -> ("Traction reciepe.Ball Load (N)"=w27:refnum<vi>)
      n217 = Unbundle By Name(w4) -> ("Traction reciepe.Lubricant Name"=w30:refnum<vi>)
      n218 = Unbundle By Name(w4) -> ("Traction reciepe.Profile File Name"=w33:refnum<vi>)
      n219 = property class="Str"(reference=w46, "Visible"=FALSE) -> (reference out=w47:refnum<vi>, error out=w45:errorcluster)  [unwired: 1 in]
      n220 = property class="MCListbox (strict)"(reference=w49, "Visible"=FALSE) -> (reference out=w48:refnum<vi>, error out=w50:errorcluster)  [unwired: 1 in]
      n221 = property class="DigNum (strict)"(reference=w52, "Visible"=FALSE) -> (reference out=w53:refnum<vi>, error out=w51:errorcluster)  [unwired: 1 in]
      n222 = property class="DigNum (strict)"(reference=w44, "Visible"=FALSE) -> (reference out=w39:refnum<vi>, error out=w43:errorcluster)  [unwired: 1 in]
      n223 = property class="DigNum (strict)"(reference=w41, "Visible"=FALSE) -> (reference out=w40:refnum<vi>, error out=w42:errorcluster)  [unwired: 1 in]
      n224 = property class="Str"(reference=w38, "Visible"=FALSE) -> (reference out=w36:refnum<vi>, error out=w37:errorcluster)  [unwired: 1 in]
      n225 = property class="DigNum (strict)"(reference=w61, "Visible"=FALSE) -> (reference out=w63:refnum<vi>, error out=w62:errorcluster)  [unwired: 1 in]
      n226 = property class="Str"(reference=w25, "Visible"=FALSE) -> (reference out=w24:refnum<vi>, error out=w26:errorcluster)  [unwired: 1 in]
      n227 = property class="DigNum (strict)"(reference=w22, "Visible"=FALSE) -> (reference out=w23:refnum<vi>, error out=w21:errorcluster)  [unwired: 1 in]
      n228 = property class="Str"(reference=w19, "Visible"=FALSE) -> (reference out=w18:refnum<vi>, error out=w20:errorcluster)  [unwired: 1 in]
      n229 = property class="Str"(reference=w27, "Visible"=FALSE) -> (reference out=w32:refnum<vi>, error out=w28:errorcluster)  [unwired: 1 in]
      n230 = property class="Str"(reference=w30, "Visible"=FALSE) -> (reference out=w31:refnum<vi>, error out=w29:errorcluster)  [unwired: 1 in]
      n231 = property class="Str"(reference=w33, "Visible"=FALSE) -> (reference out=w35:refnum<vi>, error out=w34:errorcluster)  [unwired: 1 in]
      n232 = Close Reference(reference=w47, error in (no error)=w45) -> ()  [unwired: 1 out]
      n233 = Close Reference(reference=w48, error in (no error)=w50) -> ()  [unwired: 1 out]
      n234 = Close Reference(reference=w53, error in (no error)=w51) -> ()  [unwired: 1 out]
      n235 = Close Reference(reference=w39, error in (no error)=w43) -> ()  [unwired: 1 out]
      n236 = Close Reference(reference=w40, error in (no error)=w42) -> ()  [unwired: 1 out]
      n237 = Close Reference(reference=w36, error in (no error)=w37) -> ()  [unwired: 1 out]
      n238 = Close Reference(reference=w63, error in (no error)=w62) -> ()  [unwired: 1 out]
      n239 = Close Reference(reference=w24, error in (no error)=w26) -> ()  [unwired: 1 out]
      n240 = Close Reference(reference=w23, error in (no error)=w21) -> ()  [unwired: 1 out]
      n241 = Close Reference(reference=w18, error in (no error)=w20) -> ()  [unwired: 1 out]
      n242 = Close Reference(reference=w32, error in (no error)=w28) -> ()  [unwired: 1 out]
      n243 = Close Reference(reference=w31, error in (no error)=w29) -> ()  [unwired: 1 out]
      n244 = Close Reference(reference=w35, error in (no error)=w34) -> ()  [unwired: 1 out]
      n245 = Unbundle By Name(w4) -> ("Environmental control.Acoustic Emission 3"=w9:refnum<vi>)
      n246 = Unbundle By Name(w4) -> ("Acquostic.Gains"=w8:refnum<vi>)
      n247 = property class="RadioBtnsControl (strict)"(reference=w8, "Visible"=FALSE) -> (reference out=w3:refnum<vi>, error out=w7:errorcluster)  [unwired: 1 in]
      n248 = property class="Bool (strict)"(reference=w9, "Value"=FALSE ("Visible")) -> (reference out=w11:refnum<vi>, error out=w10:errorcluster)  [unwired: 1 in]
      n249 = Close Reference(reference=w3, error in (no error)=w7) -> ()  [unwired: 1 out]
      n250 = Close Reference(reference=w11, error in (no error)=w10) -> ()  [unwired: 1 out]
    }
    frame Error {
    }
  }
